vi "Configure Output-CONTINOUS 3 channels CH 2.vi"(0 "VISA resource name":refnum<visa-resource-name>, 1 "Channel (1:3)":u16(ring)=1 items=["1"=1, "2"=2, "3"=3], 4 "Voltage Level (0.0 V)":dbl format="%.3g", 5 "error in (no error)":errorcluster, 6 "Enable Channel Output (F: False)":bool) -> (14 "VISA resource name out":refnum<visa-resource-name>, 19 "error out":errorcluster)   [LabVIEW 2017]
doc: "Configures output voltage level output and output state of the selected channel."
uses:
  <instrlib>/BK Precision 913XX/BK Precision 913XX.lvlib
panel:
  in  "Enable Channel Output (F: False) 3":bool
  in  "Voltage Level (0.0 V) 3":dbl format="%.3g"
  in  "Enable Channel Output (F: False) 2":bool
  in  "Voltage Level (0.0 V) 2":dbl format="%.3g"
  # "V"
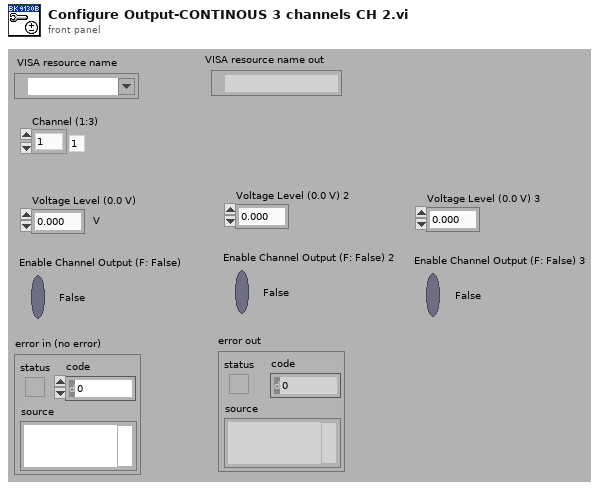
[diagram p1: front panel]
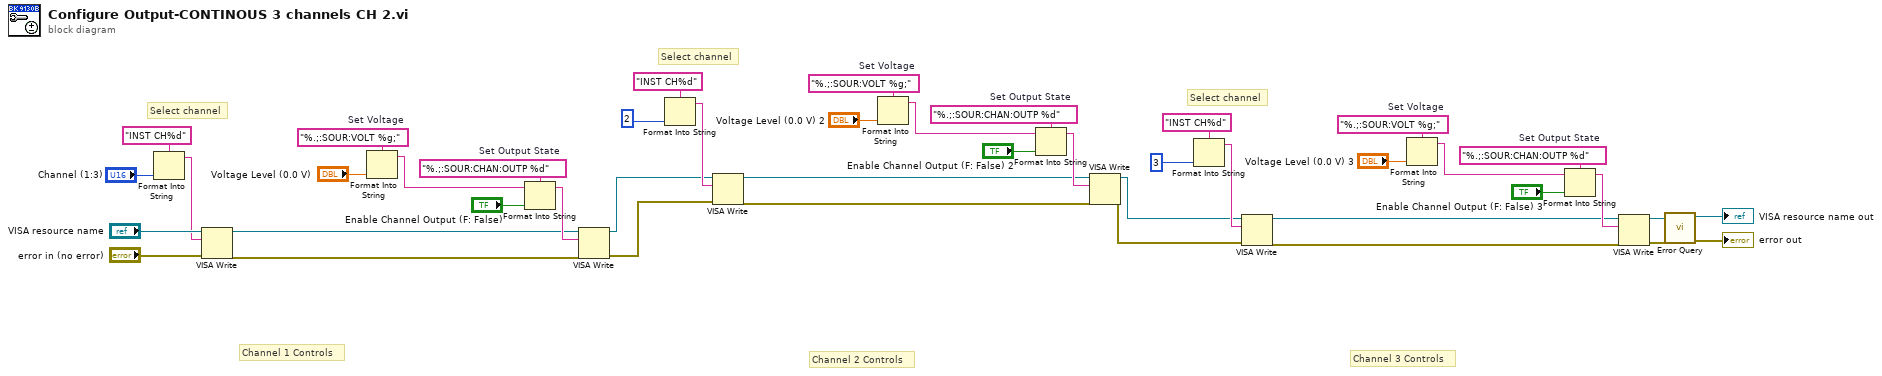
[diagram p0: block diagram]
diagram:
  w17 = "%.;:SOUR:CHAN:OUTP %d"  # Set Output State
  w19 = "%.;:SOUR:VOLT %g;"  # Set Voltage
  w27 = "%.;:SOUR:CHAN:OUTP %d"  # Set Output State
  w29 = "%.;:SOUR:VOLT %g;"  # Set Voltage
  w39 = "%.;:SOUR:CHAN:OUTP %d"  # Set Output State
  w41 = "%.;:SOUR:VOLT %g;"  # Set Voltage
  # "Channel 3 Controls"
  # "Channel 2 Controls"
  # "Channel 1 Controls"
  # "Select channel"
  # "Select channel"
  # "Select channel"
  n1 = Format Into String(format string="INST CH%d", "Channel (1:3)") -> (resulting string=w30:string)  [unwired: 2 in, 1 out]
  n2 = VISA Write(VISA resource name="VISA resource name", write buffer=w30, error in (no error)="error in (no error)") -> (VISA resource name out=w34:refnum<visa-resource-name>, error out=w33:errorcluster)  [unwired: 1 out]
  n3 = Format Into String(format string=w41, "Voltage Level (0.0 V)") -> (resulting string=w32:string)  [unwired: 2 in, 1 out]
  n4 = Format Into String(format string=w39, initial string=w32, "Enable Channel Output (F: False)") -> (resulting string=w37:string)  [unwired: 1 in, 1 out]
  n5 = VISA Write(VISA resource name=w34, write buffer=w37, error in (no error)=w33) -> (VISA resource name out=w9:refnum<visa-resource-name>, error out=w8:errorcluster)  [unwired: 1 out]
  n6 = Format Into String(format string="INST CH%d", 2) -> (resulting string=w20:string)  [unwired: 2 in, 1 out]
  n7 = VISA Write(VISA resource name=w9, write buffer=w20, error in (no error)=w8) -> (VISA resource name out=w24:refnum<visa-resource-name>, error out=w23:errorcluster)  [unwired: 1 out]
  n8 = Format Into String(format string=w29, "Voltage Level (0.0 V) 2") -> (resulting string=w22:string)  [unwired: 2 in, 1 out]
  n9 = Format Into String(format string=w27, initial string=w22, "Enable Channel Output (F: False) 2") -> (resulting string=w25:string)  [unwired: 1 in, 1 out]
  n10 = VISA Write(VISA resource name=w24, write buffer=w25, error in (no error)=w23) -> (VISA resource name out=w7:refnum<visa-resource-name>, error out=w6:errorcluster)  [unwired: 1 out]
  n11 = Format Into String(format string="INST CH%d", 3) -> (resulting string=w10:string)  [unwired: 2 in, 1 out]
  n12 = VISA Write(VISA resource name=w7, write buffer=w10, error in (no error)=w6) -> (VISA resource name out=w14:refnum<visa-resource-name>, error out=w13:errorcluster)  [unwired: 1 out]
  n13 = Format Into String(format string=w19, "Voltage Level (0.0 V) 3") -> (resulting string=w12:string)  [unwired: 2 in, 1 out]
  n14 = Format Into String(format string=w17, initial string=w12, "Enable Channel Output (F: False) 3") -> (resulting string=w15:string)  [unwired: 1 in, 1 out]
  n15 = VISA Write(VISA resource name=w14, write buffer=w15, error in (no error)=w13) -> (VISA resource name out=w5:refnum<visa-resource-name>, error out=w4:errorcluster)  [unwired: 1 out]
  n16 = call <instrlib>:"Error Query.vi"("error in (no error)"=w4, "VISA resource name"=w5) -> ("error out"=→"error out":errorcluster, "VISA resource name out"=→"VISA resource name out":refnum<visa-resource-name>)  [unwired: 6 in, 2 out]
